vi "Host-Send-Data.vi"(8 "error in\n(no error)":errorcluster, 10 "FPGA VI Reference In":refnum<k20>, 11 "Byte Stream\nFile in":refnum<file>) -> (0 "error out":errorcluster, 3 "FPGA VI Reference Out":refnum<k20>)   [LabVIEW 2016]
uses:
  <vilib>/Utility/error.llb/Error Cluster From Error Code.vi
  <vilib>/rvi/errors/niLvFpgaAdjustHostInterfaceError.vi
  <vilib>/rvi/interface/nirviMethod/nirviMethod.xnode
  <vilib>/FPGAPlugInAG/Dynamic/niLvFpga_WriteFifo_Dynamic.vi
  <vilib>/rvi/errors/niLvFpgaMergeErrorWithErrorCode.vi
panel:
  out "data":u8[](array[numeric]) format="%.0x"
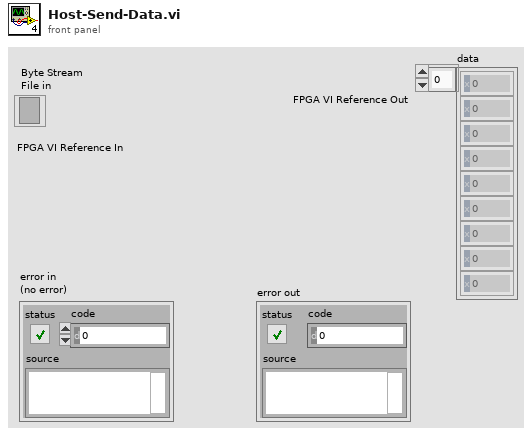
[diagram p1: front panel]
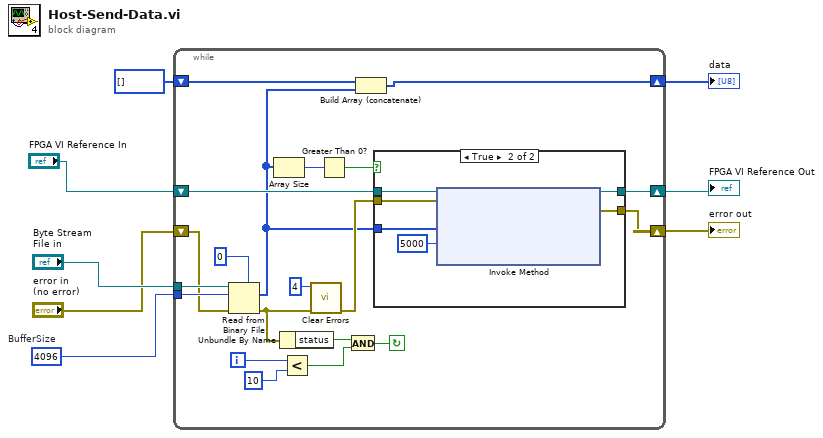
[diagram p0: block diagram]
diagram:
  w7 = 4096  # BufferSize
  n1 = while {
    tunnel: "Byte Stream\nFile in" -> [w28]
    tunnel: w7 -> [w27]
    shift-right: [w20] -> w2
    shift-left: "FPGA VI Reference In" -> [w21]
    shift-right: [w19] -> w1
    shift-left: "error in\n(no error)" -> [w17]
    shift-right: [w10] -> w4
    shift-left: u8[] [] -> [w9]
    i -> [w25]
    stop <- w26 continue-if-true
    n2 = Read from Binary File(5:u8 0 ("data type"), 8:w17, 10:w27, 11:w28) -> (0:w16:errorcluster, 2:w11:u8[])  [unwired: 2 in, 2 out]
    n3 = Array Size(array=w11) -> (size(s)=w15:i32)
    n4 = Unbundle By Name(w16) -> ("status"=w22:bool)
    n5 = Less?(x=w25, y=10) -> (x < y?=w23:bool)
    n6 = call <vilib>:"Clear Errors.vi"("error in (no error)"=w16, "specific error code to clear (0: all)"=4) -> ("error out"=w13:errorcluster)  [unwired: 4 in, 1 out]
    n7 = Greater Than 0?(x=w15) -> (x > 0?=w14:bool)
    n8 = And(x=w22, y=w23) -> (x .and. y?=w26:bool)
    n9 = Build Array (concatenate)(w9, w11) -> (w10:u8[])
    n10 = case shown="True" w14 {
      tunnel: w21 -> [w30 w36]
      tunnel: [w30 w35] -> w20
      tunnel: [w29 w34] -> w19
      tunnel: w13 -> [w29 w32]
      tunnel: w11 -> [_ w31]
      frame False {
      }
      frame True {
        n11 = xnode "Invoke Method"("FPGA VI Reference In"=w36, "error in"=w32, "Data"=w31, "Timeout (ms)"=5000) -> ("FPGA VI Reference Out"=w35:refnum<k20>, "error out"=w34:errorcluster)  [unwired: 1 out]
      }
    }
  }
  "FPGA VI Reference Out" <- w2
  "error out" <- w1
  "data" <- w4
